vi "Scale Circle for Plot XY.vi"(9 "y scale factors":cluster{"a":dbl, "b":dbl, "log?":bool} {"b" format="%.2f"; "a" format="%.2f"}, 10 "x scale factors":cluster{"a":dbl, "b":dbl, "log?":bool} {"b" format="%.2f"; "a" format="%.2f"}, 11 "circles":cluster{"x":dbl, "y":dbl, "radius":i32}[](array[cluster]) {"y" format="%.2f"; "x" format="%.2f"}) -> (3 "rectangles":cluster{i16, i16, i16, i16}[](array[cluster]))   [LabVIEW 2017]
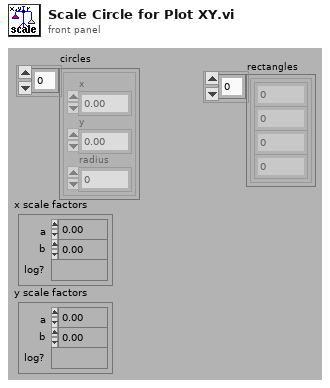
[diagram p1: front panel]
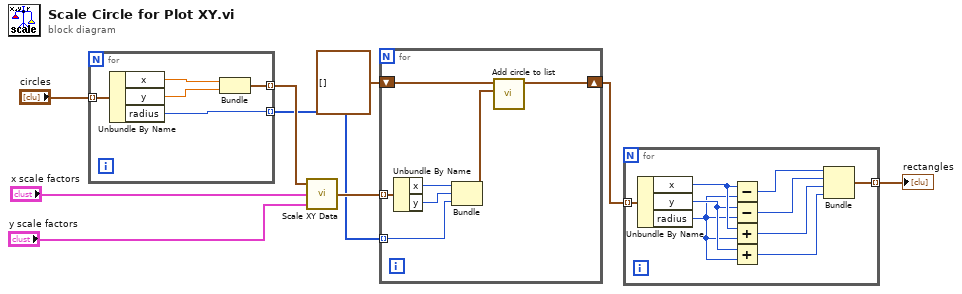
[diagram p0: block diagram]
diagram:
  n1 = for {
    tunnel: "circles" -> [w14] mode=indexing
    tunnel: [w13] -> w5 mode=indexing
    tunnel: [w10] -> w3 mode=indexing
    n2 = Unbundle By Name(w14) -> ("x"=w12:dbl, "y"=w11:dbl, "radius"=w10:i32)
    n3 = Bundle("x"=w12, "y"=w11) -> (w13:cluster{"x":dbl, "y":dbl})  [unwired: 1 in]
  }
  n4 = call <vilib>:"Scale XY Data.vi"("y scale factors"="y scale factors", "x scale factors"="x scale factors", "xy data"=w5) -> ("scaled xy data"=w4:cluster{"x":i16, "y":i16}[])
  n5 = for {
    tunnel: w4 -> [w21] mode=indexing
    tunnel: w3 -> [w18] mode=indexing
    shift-right: [w16] -> w2
    shift-left: cluster{"x":i16, "y":i16, "radius":i32}[] [] ("circle list out") -> [w17]
    n6 = Unbundle By Name(w21) -> ("x"=w20:i16, "y"=w19:i16)
    n7 = Bundle("x"=w20, "y"=w19, "radius"=w18) -> (w15:cluster{"x":i16, "y":i16, "radius":i32})  [unwired: 1 in]
    n8 = call <vilib>:"Add circle to list.vi"("circle"=w15, "circle list"=w17) -> ("circle list out"=w16:cluster{"x":i16, "y":i16, "radius":i32}[])  [unwired: 9 in]
  }
  n9 = for {
    tunnel: w2 -> [w30] mode=indexing
    tunnel: [w23] -> w6 mode=indexing
    n10 = Unbundle By Name(w30) -> ("x"=w28:i16, "y"=w27:i16, "radius"=w22:i32)
    n11 = Subtract(x=w28, y=w22) -> (x-y=w26:i32)
    n12 = Subtract(x=w27, y=w22) -> (x-y=w25:i32)
    n13 = Add(x=w28, y=w22) -> (x+y=w24:i32)
    n14 = Add(x=w27, y=w22) -> (x+y=w29:i32)
    n15 = Bundle(w26, w25, w24, w29) -> (w23:cluster{i32, i32, i32, i32})  [unwired: 1 in]
  }
  "rectangles" <- w6
